vi "test2.vi"   [LabVIEW 2014]
doc: "This VI demonstrates an asynchronous call and forget. When this VI is run, it asynchronously calls a target VI and will not wait for the results. This VI will run to completion while the target VI continues to run.\n\nThis example uses the Start Asynchronous Call method and the Open VI Reference option 0x80.\n\nWhen running this example, notice this VI finishes execution while the target VI continues to run."
uses:
  isPlaying.vi
panel:
  # "Overview: Demonstrates the use of the call and forget option (0x80) with Asynchronous VI Calls.\nInstructions:\nRun the VI. Observe the behavior of the VI being called asynchronously, and notice that this VI stops running, even when the asynchronous VI is still running. See the block diagram for more information."
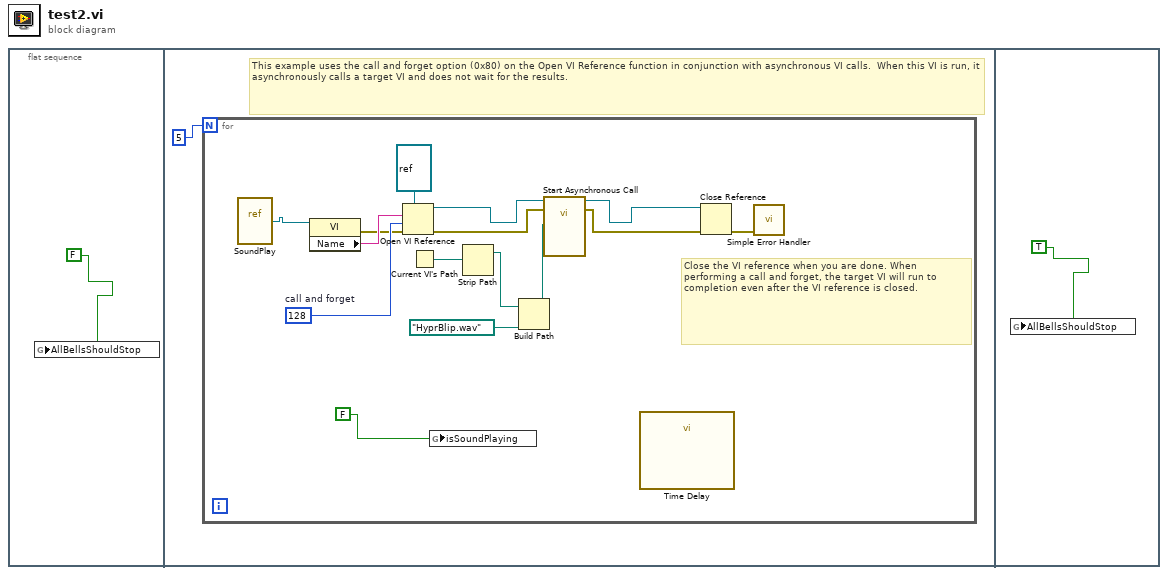
[diagram p0: block diagram]
diagram:
  n1 = flat-sequence {
    frame #0 {
      n2 = global write "isPlaying.vi" "AllBellsShouldStop"(FALSE) -> ()
    }
    frame #1 {
      # "This example uses the call and forget option (0x80) on the Open VI Reference function in conjunction with asynchronous VI calls.  When this VI is run, it asynchronously calls a target VI and does not wait for the results."
      n3 = for {
        N: 5 -> [_]
        w17 = 128  # call and forget
        # "Close the VI reference when you are done. When performing a call and forget, the target VI will run to completion even after the VI reference is closed."
        n4 = vi-ref "SoundPlay.vi"() -> (w12:refnum<vi>)
        n5 = property class="VI"(reference=w12) -> (error out=w14:errorcluster, "Name"=w15:string)  [unwired: 1 in, 1 out]
        n6 = Open VI Reference(type specifier VI Refnum (for type only)=refnum<vi> refnum, vi path=w15, options=w17, error in (no error)=w14) -> (vi reference=w11:refnum<vi>, error out=w10:errorcluster)  [unwired: 2 in]
        n7 = Current VI's Path() -> (path=w6:path)
        n8 = global write "isPlaying.vi" "isSoundPlaying"(FALSE) -> ()
        n9 = Strip Path(path=w6) -> (stripped path=w5:path)  [unwired: 1 out]
        n10 = Build Path(base path=w5, name or relative path=path "HyprBlip.wav") -> (appended path=w4:path)
        n11 = call-by-ref "Start Asynchronous Call"(reference=w11, error in=w10, "Path to Sound file"=w4) -> (reference out=w8:refnum<vi>, error out=w9:errorcluster)  [unwired: 2 in, 1 out]
        n12 = call "Time Delay"() -> ()  [unwired: 11 in, 1 out]
        n13 = Close Reference(reference=w8, error in (no error)=w9) -> (error out=w16:errorcluster)
        n14 = call <vilib>:"Simple Error Handler.vi"("error in (no error)"=w16) -> ()  [unwired: 4 in, 5 out]
      }
    }
    frame #2 {
      n15 = global write "isPlaying.vi" "AllBellsShouldStop"(TRUE) -> ()
    }
  }
